vi "Aiming Mechanism Test.vi"(10 "progress":string, 11 "progressText":string) -> (3 "endTestText":string)   [LabVIEW 2012]
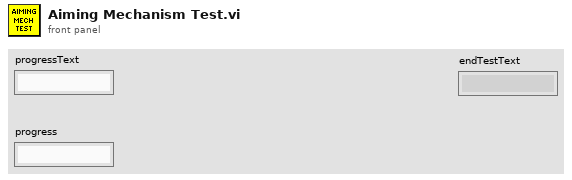
[diagram p1: front panel]
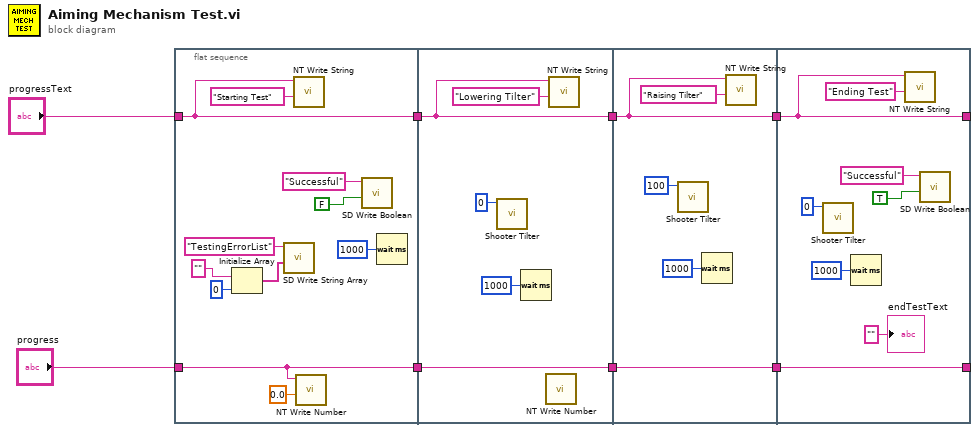
[diagram p0: block diagram]
diagram:
  n1 = flat-sequence {
    tunnel: "progressText" -> [w11]
    tunnel: "progress" -> [w10]
    tunnel: [w11] -> w6
    tunnel: [w10] -> w5
    tunnel: w6 -> [w20]
    tunnel: w5 -> [w24]
    tunnel: [w20] -> w4
    tunnel: [w24] -> w3
    tunnel: w4 -> [w25]
    tunnel: w3 -> [w29]
    tunnel: [w25] -> w2
    tunnel: [w29] -> w1
    tunnel: [w37] -> _
    tunnel: [w35] -> _
    tunnel: w2 -> [w35]
    tunnel: w1 -> [w37]
    frame #0 {
      n2 = Initialize Array("", 0 ("dimension size")) -> (w14:string[])
      n3 = call <vilib>:"SD Write String Array.vi"("String Array"=w14, "Name"="TestingErrorList") -> ()  [unwired: 8 in, 2 out]
      n4 = call <vilib>:"NT Write String.vi"("String"="Starting Test", "Name"=w11) -> ()  [unwired: 9 in, 1 out]
      n5 = call <vilib>:"NT Write Number.vi"("Numeric"=0.0, "Name"=w10) -> ()  [unwired: 9 in, 1 out]
      n6 = call <vilib>:"SD Write Boolean.vi"("Boolean"=FALSE, "Name"="Successful") -> ()  [unwired: 8 in, 2 out]
      n7 = Wait (ms)(milliseconds to wait=u32 1000) -> ()  [unwired: 1 out]
    }
    frame #1 {
      n8 = call "Shooter Tilter.vi"("numericInput"=0) -> ()  [unwired: 11 in]
      n9 = Wait (ms)(milliseconds to wait=u32 1000) -> ()  [unwired: 1 out]
      n10 = call <vilib>:"NT Write Number.vi"() -> ()  [unwired: 11 in, 1 out]
      n11 = call <vilib>:"NT Write String.vi"("String"="Lowering Tilter", "Name"=w20) -> ()  [unwired: 9 in, 1 out]
    }
    frame #2 {
      n12 = call "Shooter Tilter.vi"("numericInput"=100) -> ()  [unwired: 11 in]
      n13 = Wait (ms)(milliseconds to wait=u32 1000) -> ()  [unwired: 1 out]
      n14 = call <vilib>:"NT Write String.vi"("String"="Raising Tilter", "Name"=w25) -> ()  [unwired: 9 in, 1 out]
    }
    frame #3 {
      n15 = call "Shooter Tilter.vi"("numericInput"=0) -> ()  [unwired: 11 in]
      n16 = Wait (ms)(milliseconds to wait=u32 1000) -> ()  [unwired: 1 out]
      n17 = call <vilib>:"NT Write String.vi"("String"="Ending Test", "Name"=w35) -> ()  [unwired: 9 in, 1 out]
      n18 = call <vilib>:"SD Write Boolean.vi"("Boolean"=TRUE, "Name"="Successful") -> ()  [unwired: 8 in, 2 out]
      "endTestText" <- "" ("endTestText")
    }
  }
